vi "iRobot UART Open.vi"(8 "error in (no error)":errorcluster, 9 "Baud Rate (BPS)":T1=enum."57600", 11 "UART port in":T2) -> (0 "error out":errorcluster, 3 "UART port out":T2)   [LabVIEW 2014]
doc: "Opens a UART session with an iRobot."
uses:
  iRobot UART Port Type.ctl
  Command/Baud.ctl
  <vilib>/Instr/_visa.llb/VISA Configure Serial Port (Instr).vi
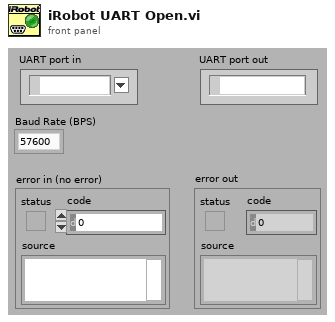
[diagram p1: front panel]
types:
  T1 = typedef "Baud.ctl" = enum8{"300", "600", "1200", "2400", "4800", "9600", "14400", "19200", "28800", "38400", "57600", "115200"}
  T2 = typedef "iRobot UART Port Type.ctl" = refnum<visa-resource-name>
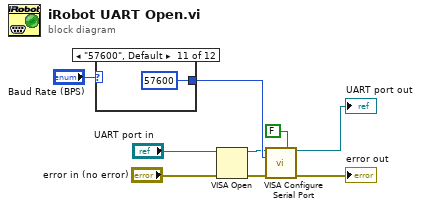
[diagram p0: block diagram]
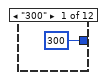
[diagram p2: hidden frame]
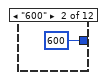
[diagram p3: hidden frame]
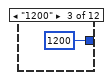
[diagram p4: hidden frame]
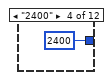
[diagram p5: hidden frame]
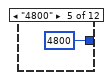
[diagram p6: hidden frame]
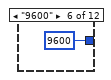
[diagram p7: hidden frame]
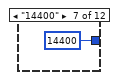
[diagram p8: hidden frame]
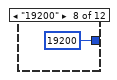
[diagram p9: hidden frame]
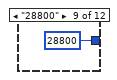
[diagram p10: hidden frame]
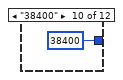
[diagram p11: hidden frame]
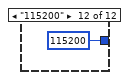
[diagram p12: hidden frame]
diagram:
  n1 = case shown="\"57600\", Default" "Baud Rate (BPS)" {
    tunnel: [u32 300 ("baud rate") u32 600 ("baud rate") u32 1200 ("baud rate") u32 2400 ("baud rate") u32 4800 ("baud rate") u32 9600 ("baud rate") u32 14400 ("baud rate") u32 19200 ("baud rate") u32 28800 ("baud rate") u32 38400 ("baud rate") u32 57600 ("baud rate") u32 115200 ("baud rate")] -> w5
    frame "300" {
    }
    frame "600" {
    }
    frame "1200" {
    }
    frame "2400" {
    }
    frame "4800" {
    }
    frame "9600" {
    }
    frame "14400" {
    }
    frame "19200" {
    }
    frame "28800" {
    }
    frame "38400" {
    }
    frame "57600", Default {
    }
    frame "115200" {
    }
  }
  n2 = VISA Open(error in (no error)="error in (no error)", VISA resource name="UART port in") -> (VISA resource name=w2:T2, error out=w1:errorcluster)  [unwired: 3 in]
  n3 = call-poly "VISA Configure Serial Port"("VISA resource name"=w2, "Enable Termination\nChar (T)"=FALSE ("Enable Termination\nChar (T)"), "baud rate (9600)"=w5, "error in (no error)"=w1) -> ("VISA resource name out"=→"UART port out":refnum<visa-resource-name>, "error out"=→"error out":errorcluster)  [unwired: 10 in]
